vi "Add New Escalation Details.vi"(8 "error in (no error)":errorcluster) -> (0 "error out":errorcluster)   [LabVIEW 2017]
uses:
  <vilib>/addons/database/Connection.llb/DB Tools Open Connec (Path).vi
  Globle/Current date.vi
  <vilib>/addons/database/_DB Variant To Data/Database Variant To Data.xnode
  <vilib>/addons/database/NI_Database_API.lvlib
panel:
  in  "Cancel Button - Archive":bool
  out "serial no":dbl
  in  "delete":bool
  in  "Shift":string(combo)
  out "Character Array":string[](array[string])
  out "Array":bool[](array[boolean])
  in  "Select Stakeholder":string(combo)
  in  "Submit":bool
  in  "Select Escalation Level":string(combo)
  in  "Mobile Number":string
  in  "Name":string
  # "Add New Escalation Details"
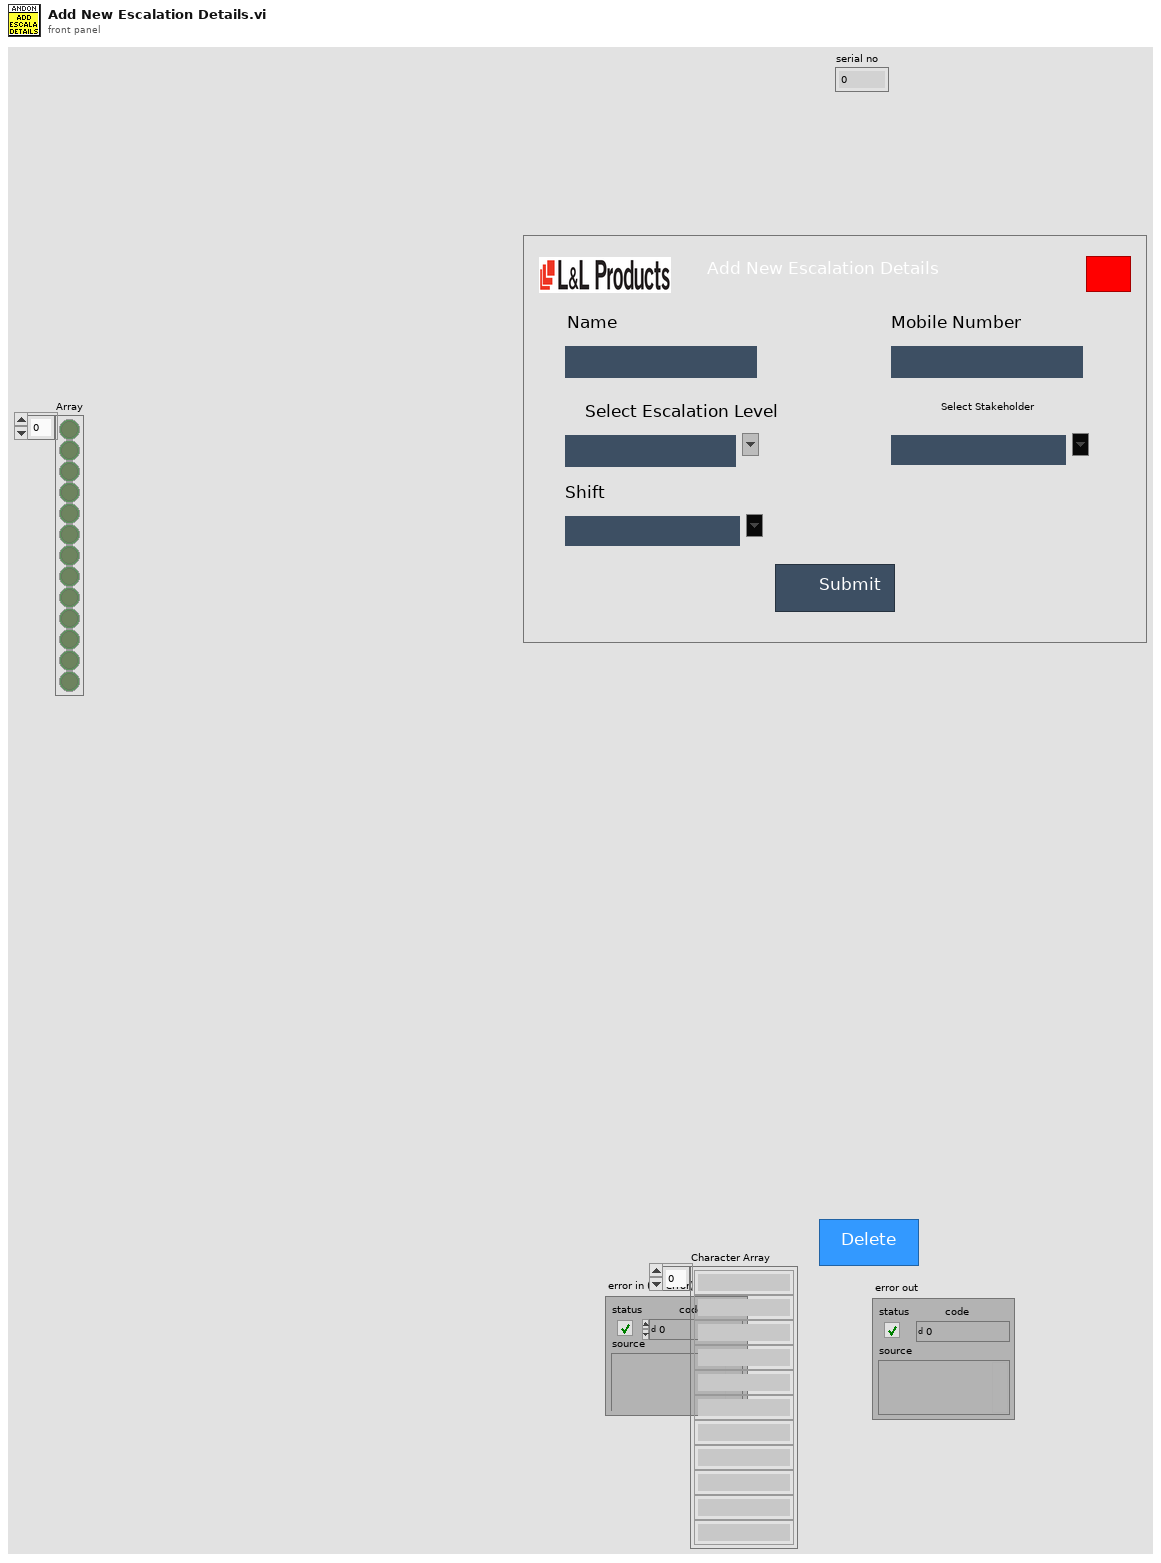
[diagram p1: front panel]
types:
  T1 = typedef "NI_Database_API.lvlib/Conn ObjectReference.ctl" = refnum<k1>
  T2 = cluster{" Name":string, string, i32, i32, "Shift":string, dbl}
  T3 = enum32{"invalid app kind", "Development System", "Run Time System", "Student Edition", "Embedded LabVIEW", "Evaluation", "Custom"}
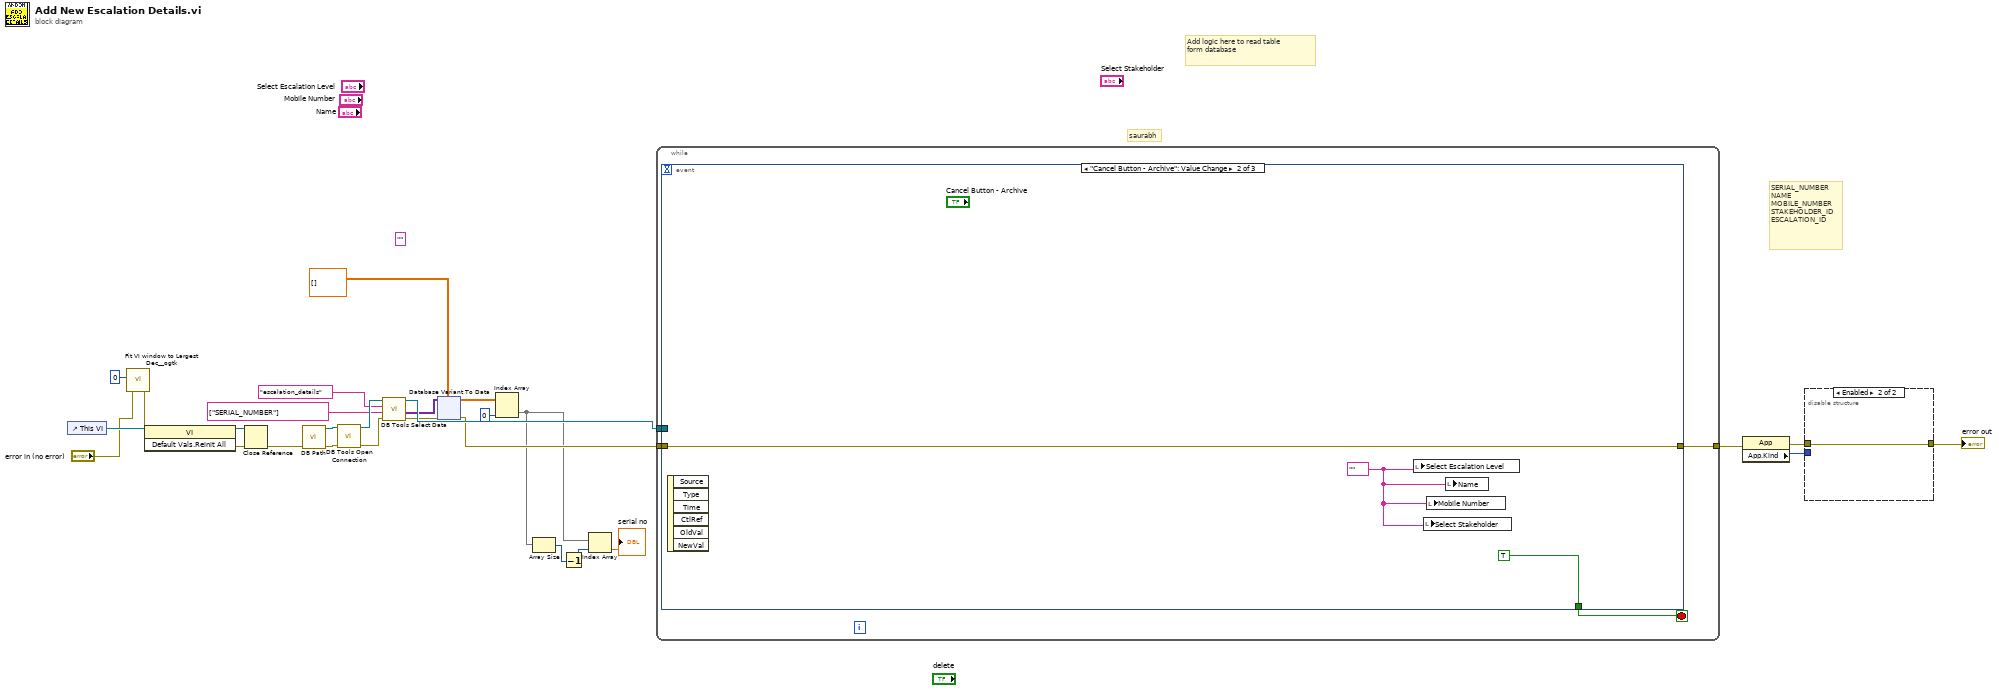
[diagram p0: block diagram]
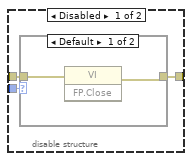
[diagram p2: hidden frame]
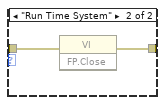
[diagram p3: hidden frame]
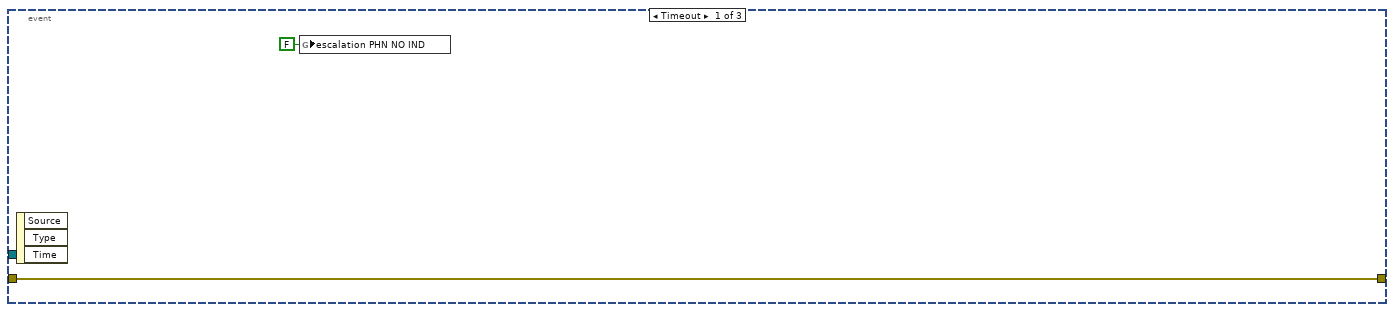
[diagram p4: hidden frame]
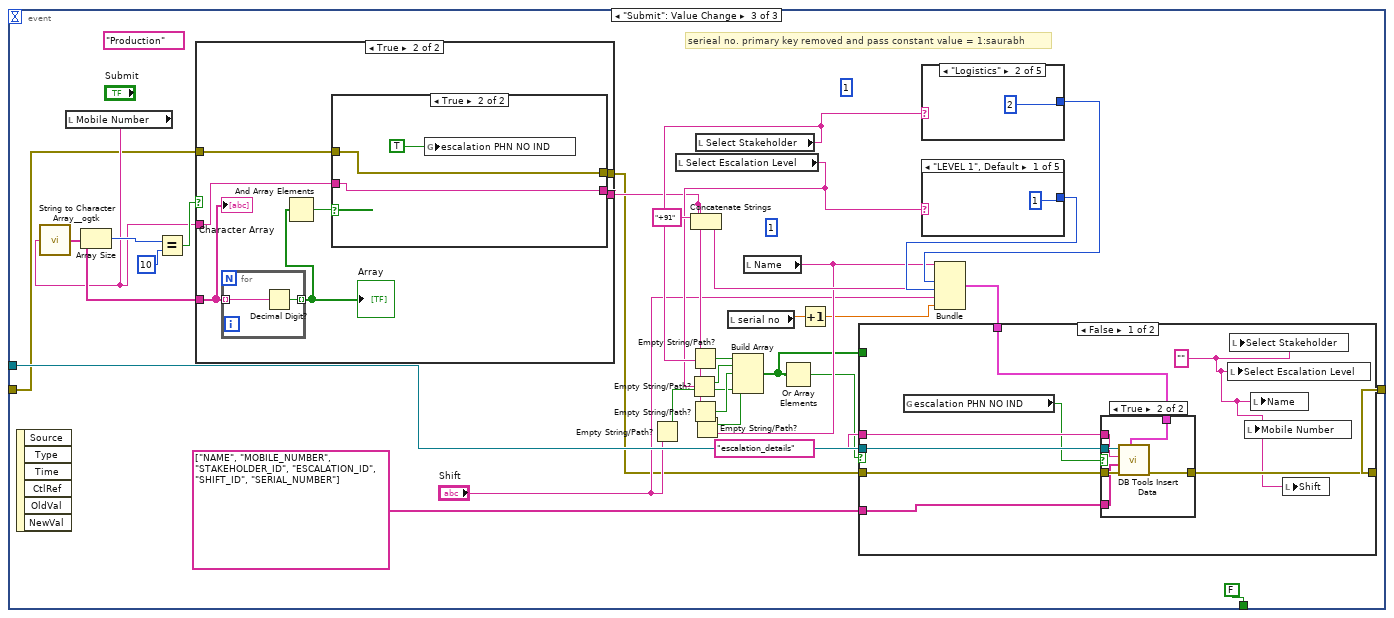
[diagram p5: hidden frame]
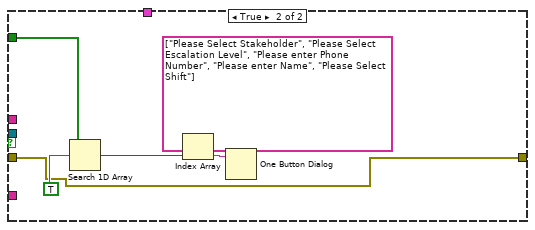
[diagram p7: hidden frame]
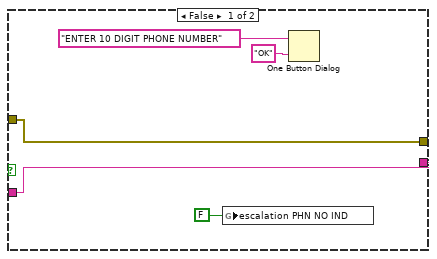
[diagram p8: hidden frame]
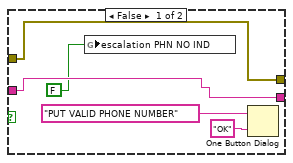
[diagram p9: hidden frame]
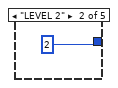
[diagram p10: hidden frame]
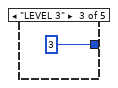
[diagram p11: hidden frame]
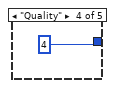
[diagram p12: hidden frame]
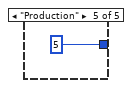
[diagram p13: hidden frame]
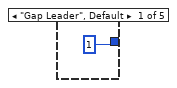
[diagram p14: hidden frame]
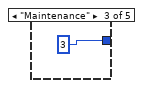
[diagram p15: hidden frame]
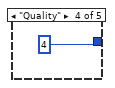
[diagram p16: hidden frame]
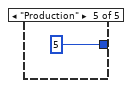
[diagram p17: hidden frame]
diagram:
  (unwired) ""
  # "saurabh"
  # "SERIAL_NUMBER\nNAME\nMOBILE_NUMBER\nSTAKEHOLDER_ID\nESCALATION_ID"
  # "Add logic here to read table\nform database"
  n1 = control-ref of="This VI"() -> (w28:refnum<vi>)
  n2 = call <userlib>:"Fit VI window to Largest Dec__ogtk.vi"("error in (no error)"="error in (no error)", "border spacing (2 px)"=0) -> ("error out"=w17:errorcluster)  [unwired: 4 in, 1 out]
  n3 = invoke class="VI" method="Default Vals.Reinit All"(reference=w28, error in=w17) -> (reference out=w26:refnum<vi>, error out=w27:errorcluster)  [unwired: 1 in, 1 out]
  n4 = Close Reference(reference=w26, error in (no error)=w27) -> (error out=w19:errorcluster)
  n5 = call "DB Path.vi"("error in"=w19) -> ("error out"=w21:errorcluster, "DB Path"=w20:path)  [unwired: 9 in]
  n6 = call-poly <vilib>:"DB Tools Open Connection.vi"("error in (no error)"=w21, "connection information"=w20) -> ("error out"=w15:errorcluster, "connection reference"=w14:T1)  [unwired: 6 in]
  n7 = call <vilib>:"DB Tools Select Data.vi"("error in (no error)"=w15, "columns"=string[] ["SERIAL_NUMBER"], "table"="escalation_details", "connection reference"=w14) -> ("error out"=w9:errorcluster, "data"=w10:variant[][], "connection reference out"=w13:T1)  [unwired: 2 in]
  n8 = xnode "Database Variant To Data"("database variant"=w10, "error in (no error)"=w9, "type"=dbl[][] []) -> ("data"=w6:dbl[][], "error out"=w8:errorcluster)
  n9 = Index Array(array=w6, index (col)=0 ("disabled index (col)")) -> (element=w2:dbl[])  [unwired: 1 in]
  n10 = Array Size(array=w2) -> (size(s)=w4:i32)
  n11 = Decrement(x=w4) -> (x-1=w3:i32)
  n12 = Index Array(array=w2, index=w3) -> (element=→"serial no":dbl)
  n13 = while {
    tunnel: w8 -> [w32]
    tunnel: [w31] -> w22
    tunnel: w13 -> [w29]
    stop <- w30 stop-if-true
    n14 = event shown="[1] \"Cancel Button - Archive\": Value Change" {
      selector: _ -> [_ _ _]
      dyn-events: _ -> [_ _ _]
      timeout: _ -> [_ _ _]
      tunnel: w32 -> [w34 w37 w41]
      tunnel: [w34 w37 w63] -> w31
      tunnel: [_ TRUE FALSE] -> w30
      tunnel: w29 -> [_ _ w67]
      event Timeout {
        n15 = event-data() -> ()  [unwired: 1 in, 3 out]
        n16 = global write "Current date.vi" "escalation PHN NO IND"(FALSE) -> ()
      }
      event "Cancel Button - Archive": Value Change {
        w35 = "" ("Select Escalation Level")
        n17 = event-data() -> ()  [unwired: 1 in, 6 out]
        n18 = local write "Select Escalation Level"(w35) -> ()
        n19 = local write "Select Stakeholder"(w35) -> ()
        n20 = local write "Mobile Number"(w35) -> ()
        n21 = local write "Name"(w35) -> ()
      }
      event "Submit": Value Change {
        (unwired) 1
        (unwired) 1
        (unwired) "Production" ("Select Stakeholder 2")
        # "serieal no. primary key removed and pass constant value = 1:saurabh"
        n22 = event-data() -> ()  [unwired: 1 in, 6 out]
        n23 = local read "Mobile Number"() -> (w56:string)
        n24 = call <userlib>:"String to Character Array__ogtk.vi"("Input String"=w56) -> ("Character Array"=w60:string[])
        n25 = Array Size(array=w60) -> (size(s)=w59:i32)
        n26 = Equal?(x=w59, y=10) -> (x = y?=w57:bool)
        n27 = case shown="True" w57 {
          tunnel: w56 -> [w91 w98]
          tunnel: w60 -> [_ w101]
          tunnel: [w91 w97] -> w51
          tunnel: [w90 w96] -> w40
          tunnel: w41 -> [w90 w95]
          frame False {
            n28 = global write "Current date.vi" "escalation PHN NO IND"(FALSE) -> ()
            n29 = One Button Dialog(message="ENTER 10 DIGIT PHONE NUMBER", button name ("OK")="OK") -> ()  [unwired: 1 out]
          }
          frame True {
            n30 = for {
              tunnel: w101 -> [w103] mode=indexing
              tunnel: [w102] -> w100 mode=indexing
              n31 = Decimal Digit?(1:w103) -> (0:w102:bool)
            }
            "Array" <- w100
            n32 = And Array Elements(Boolean array=w100) -> (logical AND=w99:bool)
            n33 = case shown="True" w99 {
              tunnel: w98 -> [w106 w111]
              tunnel: [w106 w111] -> w97
              tunnel: [w104 w109] -> w96
              tunnel: w95 -> [w104 w109]
              frame False {
                n34 = global write "Current date.vi" "escalation PHN NO IND"(FALSE) -> ()
                n35 = One Button Dialog(message="PUT VALID PHONE NUMBER", button name ("OK")="OK") -> ()  [unwired: 1 out]
              }
              frame True {
                n36 = global write "Current date.vi" "escalation PHN NO IND"(TRUE ("PHONE NUMBER IND")) -> ()
              }
            }
            "Character Array" <- w101
          }
        }
        n37 = Empty String/Path?(string/path="Shift") -> (empty?=w42:bool)
        n38 = local read "Select Escalation Level"() -> (w52:string)
        n39 = Empty String/Path?(string/path=w52) -> (empty?=w48:bool)
        n40 = Empty String/Path?(string/path=w51) -> (empty?=w47:bool)
        n41 = Concatenate Strings("+91" ("string"), w51) -> (w54:string)
        n42 = local read "Select Stakeholder"() -> (w53:string)
        n43 = Empty String/Path?(string/path=w53) -> (empty?=w49:bool)
        n44 = local read "serial no"() -> (w39:dbl)
        n45 = local read "Name"() -> (w50:string)
        n46 = Empty String/Path?(string/path=w50) -> (empty?=w46:bool)
        n47 = Build Array(w49, w48, w47, w46, w42) -> (w44:bool[])
        n48 = Or Array Elements(Boolean array=w44) -> (logical OR=w45:bool)
        n49 = Increment(x=w39) -> (x+1=w38:dbl)
        n50 = case shown="\"Logistics\"" w53 {
          tunnel: [1 2 3 4 5] -> w62
          frame "Gap Leader", Default {
          }
          frame "Logistics" {
          }
          frame "Maintenance" {
          }
          frame "Quality" {
          }
          frame "Production" {
          }
        }
        n51 = case shown="\"LEVEL 1\", Default" w52 {
          tunnel: [1 2 3 4 5] -> w61
          frame "LEVEL 1", Default {
          }
          frame "LEVEL 2" {
          }
          frame "LEVEL 3" {
          }
          frame "Quality" {
          }
          frame "Production" {
          }
        }
        n52 = Bundle("Name"=w50, w54, w62, w61, "Shift"="Shift", w38) -> (w64:T2)  [unwired: 1 in]
        n53 = case shown="False" w45 {
          tunnel: w40 -> [w76 w84]
          tunnel: w67 -> [w75 _]
          tunnel: string[] ["NAME", "MOBILE_NUMBER", "STAKEHOLDER_ID", "ESCALATION_ID", "SHIFT_ID", "SERIAL_NUMBER"] ("columns") -> [w74 _]
          tunnel: "escalation_details" ("table") -> [w73 _]
          tunnel: w64 -> [w72 _]
          tunnel: [w71 w84] -> w63
          tunnel: w44 -> [_ w85]
          frame False {
            w70 = ""
            n54 = global read "Current date.vi" "escalation PHN NO IND"() -> (w69:bool)
            n55 = case shown="True" w69 {
              tunnel: w76 -> [w77 w83]
              tunnel: w75 -> [_ w82]
              tunnel: w74 -> [_ w81]
              tunnel: w73 -> [_ w80]
              tunnel: w72 -> [_ w79]
              tunnel: [w77 w78] -> w71
              frame False {
              }
              frame True {
                n56 = call <vilib>:"DB Tools Insert Data.vi"("data"=w79, "error in (no error)"=w83, "columns"=w81, "table"=w80, "connection reference"=w82) -> ("error out"=w78:errorcluster)  [unwired: 5 in, 1 out]
              }
            }
            n57 = local write "Select Escalation Level"(w70) -> ()
            n58 = local write "Select Stakeholder"(w70) -> ()
            n59 = local write "Mobile Number"(w70) -> ()
            n60 = local write "Name"(w70) -> ()
            n61 = local write "Shift"(w70) -> ()
          }
          frame True {
            n62 = Search 1D Array(1D array=w85, element=TRUE) -> (index of element=w88:i32)  [unwired: 1 in]
            n63 = Index Array(array=string[] ["Please Select Stakeholder", "Please Select Escalation Level", "Please enter Phone Number", "Please enter Name", "Please Select Shift"], index=w88) -> (element=w86:string)
            n64 = One Button Dialog(message=w86) -> ()  [unwired: 1 in, 1 out]
          }
        }
      }
    }
  }
  n65 = property class="App"(error in=w22) -> (error out=w24:errorcluster, "App.Kind"=w25:T3)  [unwired: 1 in, 1 out]
  n66 = disable-structure shown="Enabled" {
    disable-tunnel: w25 -> [w124 _]
    disable-tunnel: w24 -> [w123 w129]
    disable-tunnel: [w122 w129] -> w23
    frame Disabled {
      n67 = case shown="Default" w124 {
        tunnel: w123 -> [w126 w128]
        tunnel: [w125 w127] -> w122
        frame Default {
          n68 = invoke class="VI" method="FP.Close"(error in=w126) -> (error out=w125:errorcluster)  [unwired: 2 in, 2 out]
        }
        frame "Run Time System" {
          n69 = invoke class="VI" method="FP.Close"(error in=w128) -> (error out=w127:errorcluster)  [unwired: 2 in, 2 out]
        }
      }
    }
    frame Enabled {
    }
  }
  "error out" <- w23
